vi "Create Link Paths.vi"(3 "Item":string, 5 "CD":string, 7 "Target":string, 9 "Measurement? (F)":bool, 10 "Canceled?":bool, 11 "Link In":T1) -> (2 "Link Out":T1)   [LabVIEW 2011]
uses:
  Controls/ECUMC Item.ctl
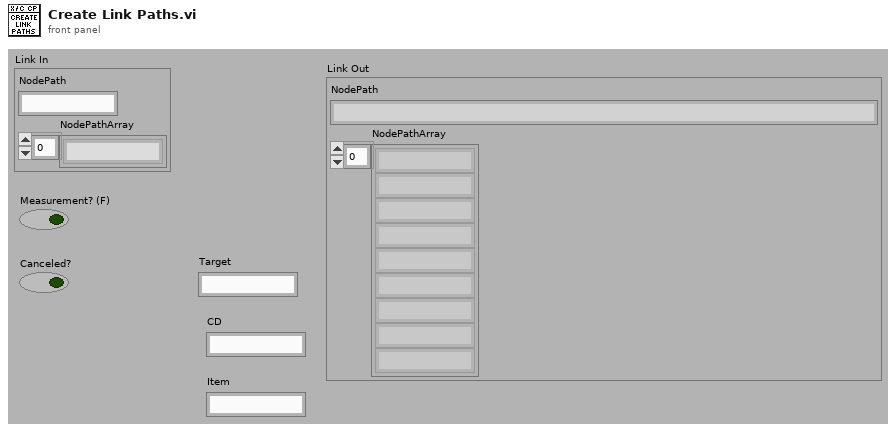
[diagram p1: front panel]
types:
  T1 = typedef "ECUMC Item.ctl" = cluster{"NodePath":string, "NodePathArray":string[]}
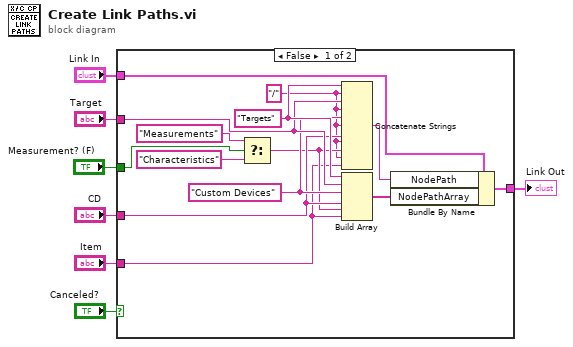
[diagram p0: block diagram]
diagram:
  n1 = case shown="False" "Canceled?" {
    tunnel: [w16 w22] -> w5
    tunnel: "Link In" -> [w18 w22]
    tunnel: "Measurement? (F)" -> [w19 _]
    tunnel: "Target" -> [w13 _]
    tunnel: "CD" -> [w11 _]
    tunnel: "Item" -> [w8 _]
    frame False {
      w9 = "/"
      w12 = "Custom Devices" ("string")
      w14 = "Targets" ("string")
      n2 = Select(t="Measurements" ("string"), s=w19, f="Characteristics" ("string")) -> (s? t:f=w10:string)
      n3 = Concatenate Strings(w14, w9, w13, w9, w12, w9, w11, w9, w10, w9, w8) -> (w17:string)
      n4 = Build Array(w14, w13, w12, w11, w10, w8) -> (w15:string[])
      n5 = Bundle By Name(cluster=w18, "NodePath"=w17, "NodePathArray"=w15) -> (w16:T1)
    }
    frame True {
    }
  }
  "Link Out" <- w5
